vi "Convert bool array to U8 Array.vi"(7 "Boolean array":bool[](array[boolean])) -> (8 "Array":u8[](array[numeric]))   [LabVIEW 2020]
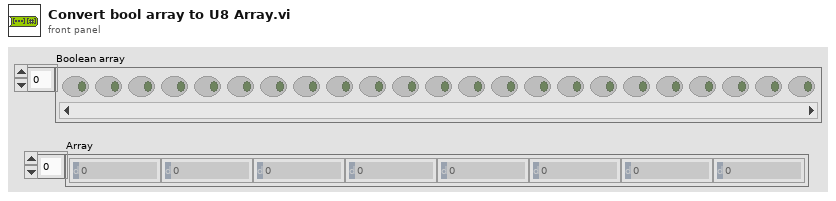
[diagram p1: front panel]
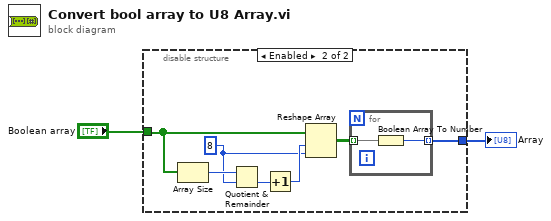
[diagram p0: block diagram]
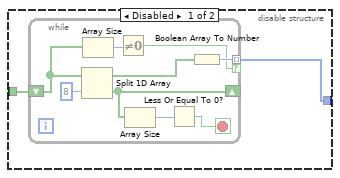
[diagram p2: hidden frame]
diagram:
  n1 = disable-structure shown="Enabled" {
    disable-tunnel: [w4 w16] -> w2
    disable-tunnel: "Boolean array" -> [w3 w20]
    frame Disabled {
      n2 = while {
        tunnel: [w12] -> w4 mode=indexing if=w5
        shift-right: [w11] -> _
        shift-left: w3 -> [w7]
        stop <- w9 stop-if-true
        n3 = Split 1D Array(array=w7, index=8) -> (first subarray=w8:bool[], second subarray=w11:bool[])
        n4 = Array Size(array=w7) -> (size(s)=w6:i32)
        n5 = Not Equal To 0?(x=w6) -> (x != 0?=w5:bool)
        n6 = Array Size(array=w11) -> (size(s)=w10:i32)
        n7 = Less Or Equal To 0?(x=w10) -> (x <= 0?=w9:bool)
        n8 = Boolean Array To Number(Boolean array=w8) -> (number=w12:u32)
      }
    }
    frame Enabled {
      w14 = 8 ("dimension size")
      n9 = Array Size(array=w20) -> (size(s)=w19:i32)
      n10 = Quotient & Remainder(x=w19, y=w14) -> (floor(x/y)=w18:i32)  [unwired: 1 out]
      n11 = Increment(x=w18) -> (x+1=w15:i32)
      n12 = Reshape Array(w20, w15, w14) -> (w17:bool[][])
      n13 = for {
        tunnel: w17 -> [w22] mode=indexing
        tunnel: [w21] -> w16 mode=indexing
        n14 = Boolean Array To Number(Boolean array=w22) -> (number=w21:u8)
      }
    }
  }
  "Array" <- w2
